vi "Gasket with or without display.vi"(6 "黑像个数":dbl, 7 "有无定位":bool, 8 "error in (no error)":errorcluster caption="错误输入（无错误）", 9 "黑像素阀值判定个数":dbl, 10 "ROI Descriptor":T2 {"Contours"."Type" items=["No Selection", "Point", "Line", "Rectangle", "Oval", "Polygon", "Freehand Region", "Annulus", "Unused2", "Unused3", "Broken Line", "Freehand Line", "Rotated Rectangle"]}, 11 "原始图像 IN":T3(plugin-control)) -> (0 "error out":errorcluster caption="错误输出", 1 "异常":bool, 2 "铜片有/无":bool, 3 "原始图像 OUT":T3(plugin-control))   [LabVIEW 2017]
panel:
  out "Annulus":T1 {"End Angle" min=-90.0 max=90.0 step=1.0 format="%.2f"; "Start Angle" min=-90.0 max=90.0 step=1.0 format="%.2f"; "Center X" scale=0.0..1024.0}
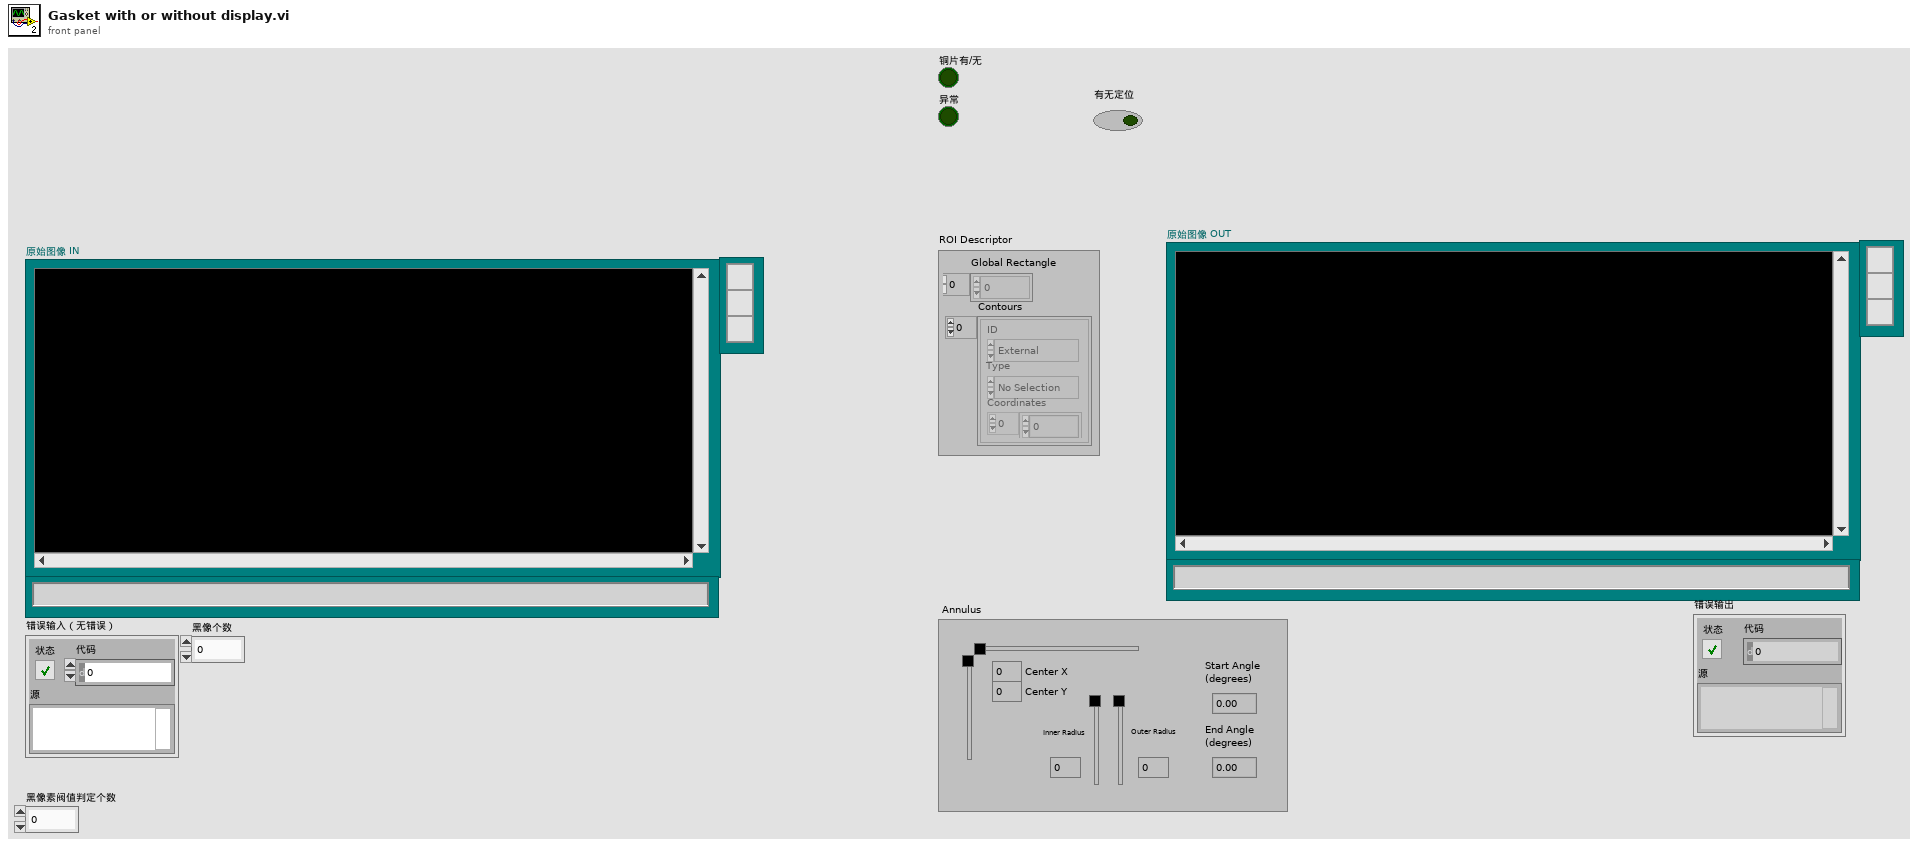
[diagram p1: front panel]
types:
  T1 = typedef "IMAQ Circle" = cluster{"Center X":i32, "Center Y":i32, "Inner Radius":i32, "Outer Radius":i32, "Start Angle":dbl, "End Angle":dbl}
  T2 = typedef "ROI Descriptor" = cluster{"Global Rectangle":i32[], "Contours":cluster{"ID":enum32{"External", "Internal"}, "Type":u32, "Coordinates":i32[]}[]}
  T3 = typedef "IMAQ Image.ctl" = refnum<image>
  T4 = cluster{"Desired Font (Application)":enum16{"User-specified Font", "Application Font", "System Font", "Dialog Font"}, "[User-specified Font]":cluster{"Font Name":string, "Size":i16, "Strikeout?":bool, "Italic?":bool, "Underline?":bool, "Outline?":bool, "Shadow?":bool, "Bold?":bool, "Rotation Angle":dbl}, "Horizontal Alignment":i16, "Vertical Alignment":i16}
  T5 = cluster{"Left":i32, "Top":i32, "rigte":i32, "bottom 3":i32}
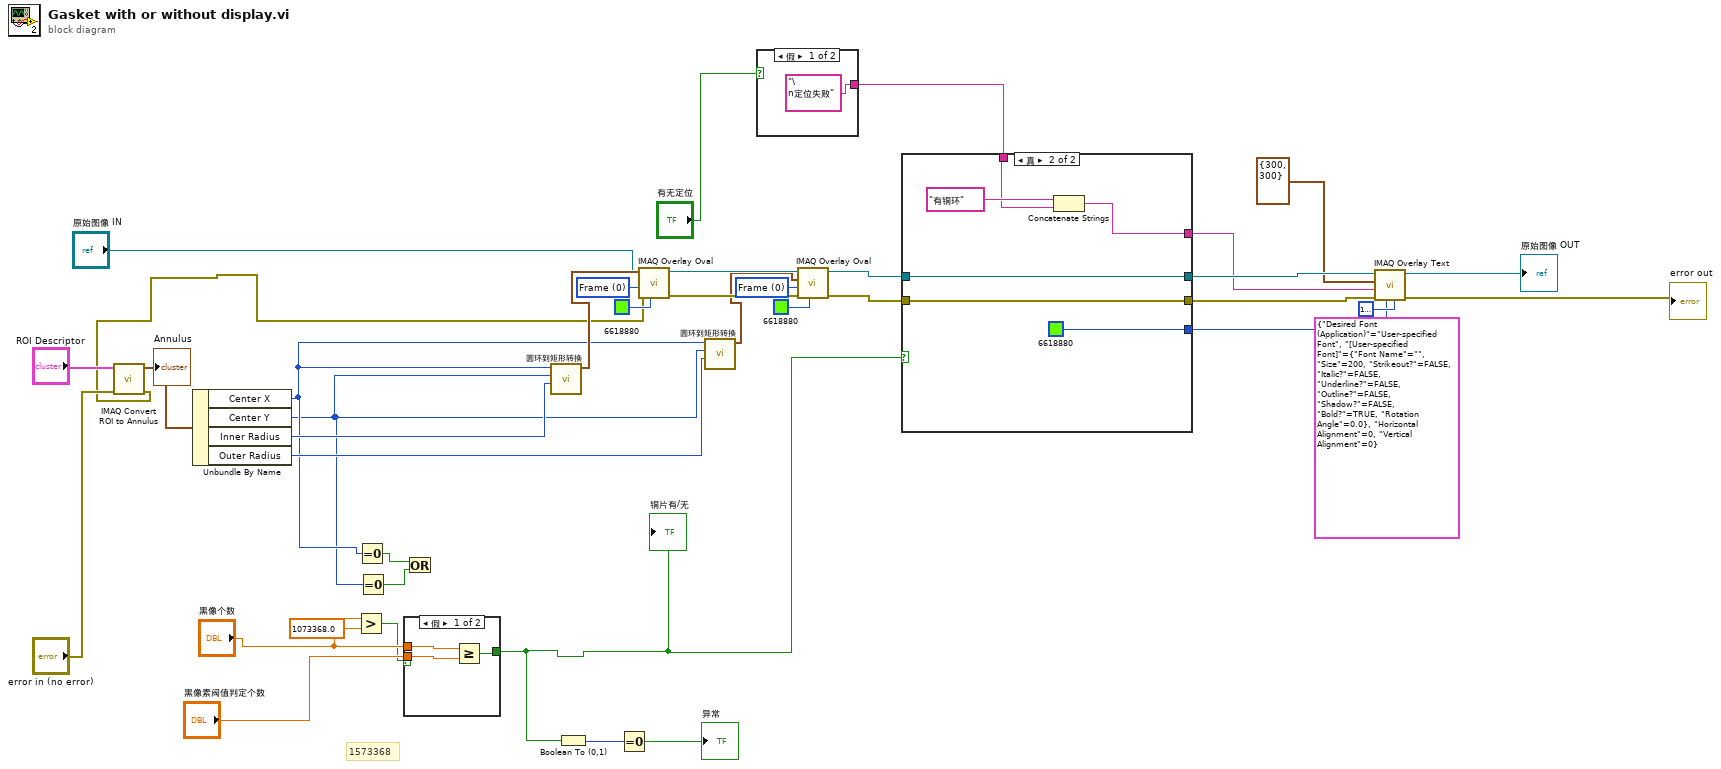
[diagram p0: block diagram]
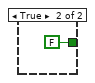
[diagram p2: hidden frame]
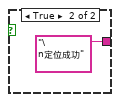
[diagram p3: hidden frame]
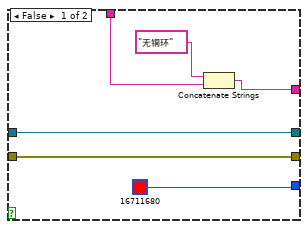
[diagram p4: hidden frame]
diagram:
  w36 = u32 0 items=["Frame", "Fill"] ("Drawing Mode (Frame)")
  w39 = u32 0 items=["Frame", "Fill"] ("Drawing Mode (Frame)")
  # "1573368"
  n1 = call "IMAQ Convert ROI to Annulus"("error in (no error)"="error in (no error)", "ROI Descriptor"="ROI Descriptor") -> ("error out"=w12:errorcluster, "Annulus"=w30:T1)  [unwired: 7 in]
  "Annulus" <- w30
  n2 = Unbundle By Name(w30) -> ("Center X"=w10:i32, "Center Y"=w9:i32, "Inner Radius"=w29:i32, "Outer Radius"=w27:i32)
  n3 = Greater?(x="黑像个数", y=1073368.0) -> (0:w1:bool)
  n4 = Equal To 0?(x=w10) -> (x = 0?=w8:bool)
  n5 = Equal To 0?(x=w9) -> (x = 0?=w7:bool)
  n6 = case shown="假" w1 {
    tunnel: "黑像素阀值判定个数" -> [w42 _]
    tunnel: [w41 FALSE] -> w6
    tunnel: "黑像个数" -> [w40 _]
    frame False {
      n7 = Greater Or Equal?(x=w40, y=w42) -> (x >= y?=w41:bool)
    }
    frame True {
    }
  }
  "铜片有/无" <- w6
  n8 = Or(x=w8, y=w7) -> ()  [unwired: 1 out]
  n9 = call "圆环到矩形转换.vi"("Radius"=w29, "CenerY"=w9, "CenerX"=w10) -> ("Bounding Rectangle out"=w31:T5)  [unwired: 8 in]
  n10 = Boolean To (0,1)(Boolean=w6) -> (0, 1=w14:i16)
  n11 = Equal To 0?(x=w14) -> (x = 0?=→"异常":bool)
  n12 = call "IMAQ Overlay Oval"("Color"=u32 6618880, "error in (no error)"=w12, "Drawing Mode (Frame)"=w39, "Bounding Rectangle"=w31, "Image"="原始图像 IN") -> ("error out"=w37:errorcluster, "Image Out"=w38:T3)  [unwired: 5 in]
  n13 = call "圆环到矩形转换.vi"("Radius"=w27, "CenerY"=w9, "CenerX"=w10) -> ("Bounding Rectangle out"=w28:T5)  [unwired: 8 in]
  n14 = case shown="假" "有无定位" {
    tunnel: ["\n定位失败" "\n定位成功"] -> w4
    frame False {
    }
    frame True {
    }
  }
  n15 = call "IMAQ Overlay Oval"("Color"=u32 6618880, "error in (no error)"=w37, "Drawing Mode (Frame)"=w36, "Bounding Rectangle"=w28, "Image"=w38) -> ("error out"=w24:errorcluster, "Image Out"=w25:T3)  [unwired: 5 in]
  n16 = case shown="真" w6 {
    tunnel: w25 -> [w51 w57]
    tunnel: w24 -> [w50 w56]
    tunnel: [w51 w57] -> w23
    tunnel: [w50 w56] -> w21
    tunnel: [w47 w53] -> w18
    tunnel: [u32 16711680 ("Text Color (black)") u32 6618880 ("Text Color (black)")] -> w16
    tunnel: w4 -> [w46 w52]
    frame False {
      n17 = Concatenate Strings("无铜环" ("String"), w46) -> (w47:string)
    }
    frame True {
      n18 = Concatenate Strings("有铜环" ("String"), w52) -> (w53:string)
    }
  }
  n19 = call "IMAQ Overlay Text"("BG Color (Transparent)"=u32 16777216, "Text Color (black)"=w16, "Font, Size & Style"=T4 {"Desired Font (Application)"=enum."User-specified Font", "[User-specified Font]"={"Font Name"="", "Size"=200, "Strikeout?"=FALSE, "Italic?"=FALSE, "Underline?"=FALSE, "Outline?"=FALSE, "Shadow?"=FALSE, "Bold?"=TRUE, "Rotation Angle"=0.0}, "Horizontal Alignment"=0, "Vertical Alignment"=0}, "error in (no error)"=w21, "String"=w18, "Origin"=cluster{"X":i32, "Y":i32} {"X"=300, "Y"=300}, "Image"=w23) -> ("error out"=→"error out":errorcluster, "Image Out"=→"原始图像 OUT":T3)  [unwired: 3 in]
